vi "ModbuswriteDriver.vi"(10 "M;otor Speed Controls":T1, 11 "Motor Bool Control":T2) -> (3 "error IO":errorcluster)   [LabVIEW 2024]
uses:
  Torsjonsrigg/support/MotorBoolControls.ctl
  Torsjonsrigg/support/MotorSpeedControls.ctl
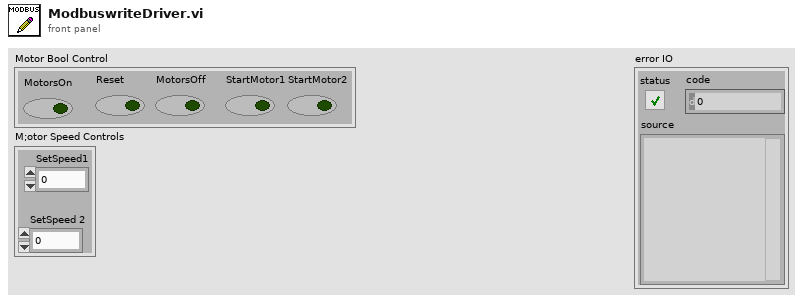
[diagram p1: front panel]
types:
  T1 = typedef "MotorSpeedControls.ctl" = cluster{"SetSpeed1":dbl, "SetSpeed 2":dbl}
  T2 = typedef "MotorBoolControls.ctl" = cluster{"MotorsOn":bool, "Reset":bool, "MotorsOff":bool, "StartMotor1":bool, "StartMotor2":bool}
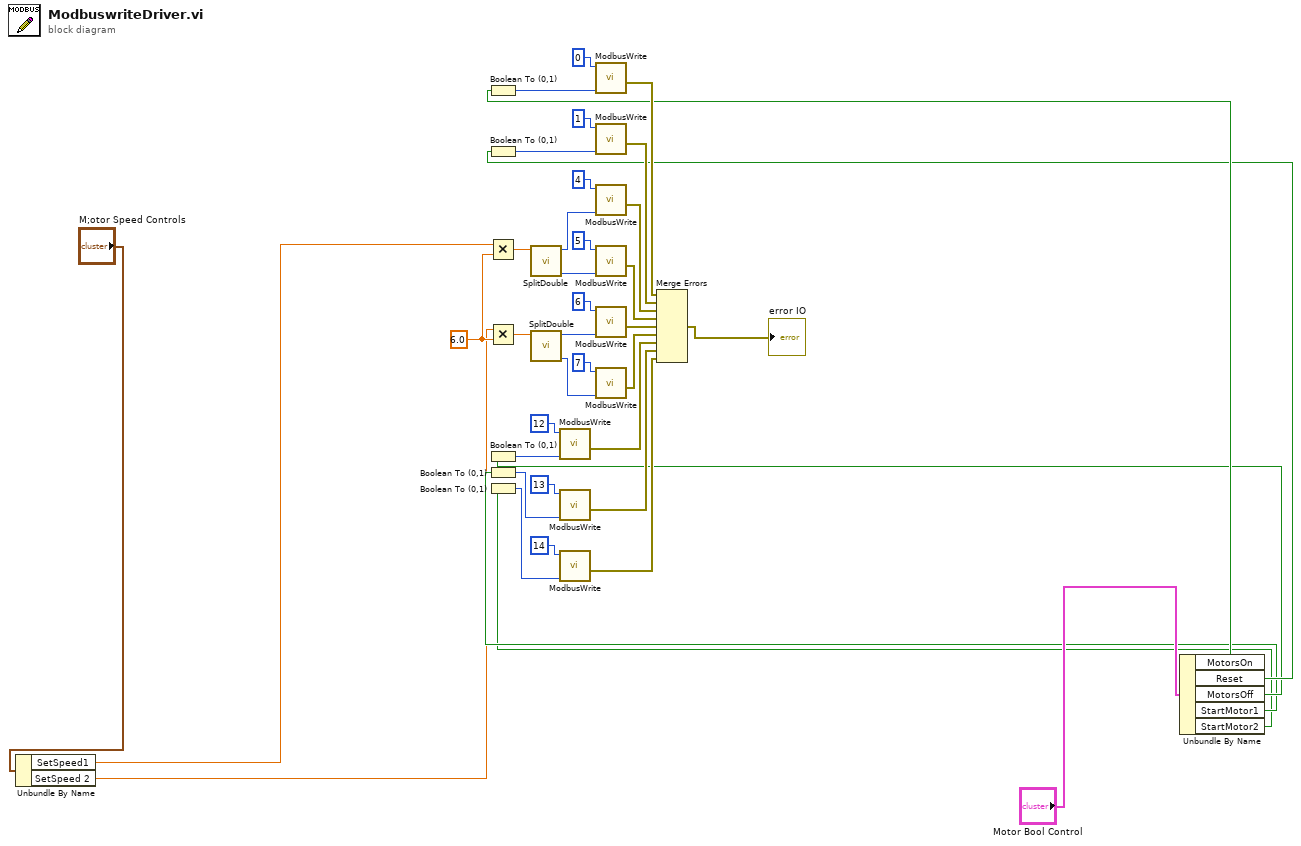
[diagram p0: block diagram]
diagram:
  w9 = 6.0 ("y")
  n1 = Unbundle By Name("M;otor Speed Controls") -> ("SetSpeed1"=w3:dbl, "SetSpeed 2"=w2:dbl)
  n2 = Multiply(x=w3, y=w9) -> (x*y=w11:dbl)
  n3 = Multiply(x=w2, y=w9) -> (x*y=w10:dbl)
  n4 = call "SplitDouble.vi"("number"=w11) -> ("Low"=w31:i16, "High"=w33:i16)  [unwired: 9 in]
  n5 = call "SplitDouble.vi"("number"=w10) -> ("Low"=w28:i16, "High"=w30:i16)  [unwired: 9 in]
  n6 = call "ModbusWrite.vi"("address"=u16 4, "holding register value"=w33) -> ("error out"=w22:errorcluster)  [unwired: 7 in]
  n7 = call "ModbusWrite.vi"("address"=u16 5, "holding register value"=w31) -> ("error out"=w21:errorcluster)  [unwired: 7 in]
  n8 = call "ModbusWrite.vi"("address"=u16 6, "holding register value"=w30) -> ("error out"=w20:errorcluster)  [unwired: 7 in]
  n9 = call "ModbusWrite.vi"("address"=u16 7, "holding register value"=w28) -> ("error out"=w19:errorcluster)  [unwired: 7 in]
  n10 = Unbundle By Name("Motor Bool Control") -> ("MotorsOn"=w8:bool, "Reset"=w7:bool, "MotorsOff"=w6:bool, "StartMotor1"=w5:bool, "StartMotor2"=w4:bool)
  n11 = Boolean To (0,1)(Boolean=w8) -> (0, 1=w34:i16)
  n12 = Boolean To (0,1)(Boolean=w7) -> (0, 1=w35:i16)
  n13 = Boolean To (0,1)(Boolean=w6) -> (0, 1=w25:i16)
  n14 = Boolean To (0,1)(Boolean=w5) -> (0, 1=w16:i16)
  n15 = Boolean To (0,1)(Boolean=w4) -> (0, 1=w14:i16)
  n16 = call "ModbusWrite.vi"("address"=u16 12, "holding register value"=w25) -> ("error out"=w18:errorcluster)  [unwired: 7 in]
  n17 = call "ModbusWrite.vi"("address"=u16 13, "holding register value"=w16) -> ("error out"=w13:errorcluster)  [unwired: 7 in]
  n18 = call "ModbusWrite.vi"("address"=u16 14, "holding register value"=w14) -> ("error out"=w12:errorcluster)  [unwired: 7 in]
  n19 = call "ModbusWrite.vi"("address"=u16 0, "holding register value"=w34) -> ("error out"=w24:errorcluster)  [unwired: 7 in]
  n20 = call "ModbusWrite.vi"("address"=u16 1, "holding register value"=w35) -> ("error out"=w23:errorcluster)  [unwired: 7 in]
  n21 = Merge Errors(w24, w23, w22, w21, w20, w19, w18, w13, w12) -> (→"error IO":errorcluster)
